vi "LOGGER Loop.vi"(8 "error in":errorcluster, 10 "Queues":T1, 11 "Notifiers":T2) -> (0 "error out":errorcluster)   [LabVIEW 2015, in "Logger.lvlib"]
uses:
  Logger.lvlib
  support/Message Queue/Message Queue.lvlib
  TypeDefs/Logger State.ctl
  TypeDefs/Logger Data.ctl
  Model/TypeDefs/Get Model Status Control.ctl
  Model/Model.lvlib
  <vilib>/ErrorRing/Error Ring.xnode
  support/Global names.vi
  <vilib>/Utility/error.llb/Error Cluster From Error Code.vi
  support/Message Queue/Message Cluster.ctl
  support/Notifiers/Notifiers.ctl
  support/Notifiers/Notifiers.lvlib
  support/Message Queue/All Message Queues.ctl
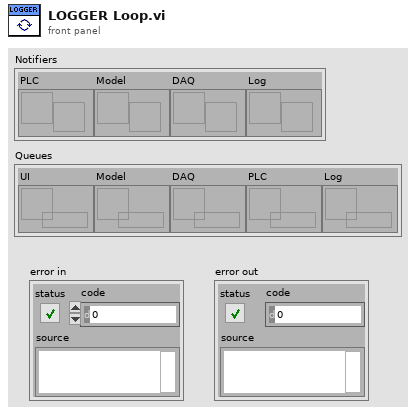
[diagram p1: front panel]
types:
  T1 = typedef "Message Queue.lvlib/All Message Queues.ctl" = cluster{"UI":refnum<queue>, "Model":refnum<queue>, "DAQ":refnum<queue>, "PLC":refnum<queue>, "Log":refnum<queue>}
  T2 = typedef "Notifiers.lvlib/Notifiers.ctl" = cluster{"PLC":refnum<notifier>, "Model":refnum<notifier>, "DAQ":refnum<notifier>, "Log":refnum<notifier>}
  T3 = typedef "Logger.lvlib/Logger Data.ctl" = cluster{"tdms file out":refnum<k34>, "State":T4, "Path":path}
  T4 = typedef "Logger.lvlib/Logger State.ctl" = enum16{"Idle", "Working"}
  T5 = enum16{"open", "open or create", "create or replace", "create", "open (read-only)"}
  T6 = typedef "Model.lvlib/Get Model Status Control.ctl" = cluster{"Position":dbl, "Pump State":bool, "Fluid Flow":dbl, "Fluid Level":dbl, "Barrel Number":i32, "Spill Alarm":bool, "Level Alarm":bool}
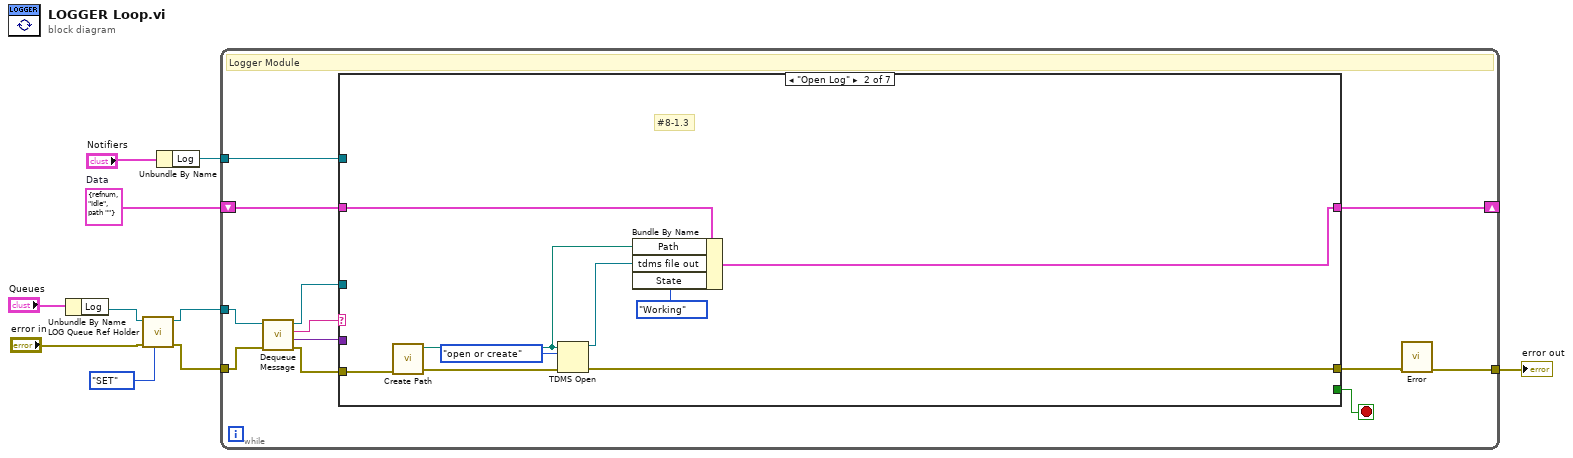
[diagram p0: block diagram]
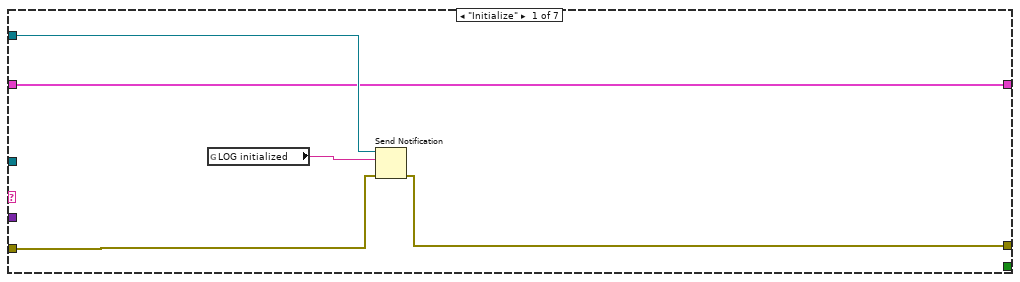
[diagram p2: hidden frame]
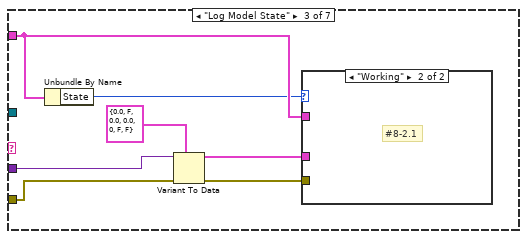
[diagram p3: hidden frame]
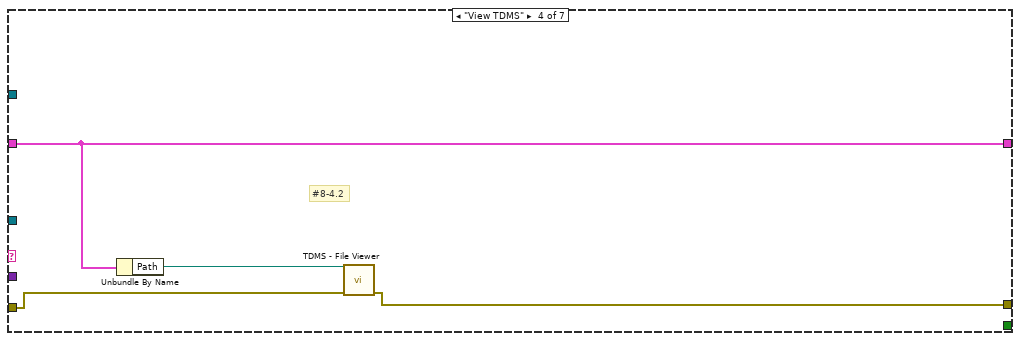
[diagram p5: hidden frame]
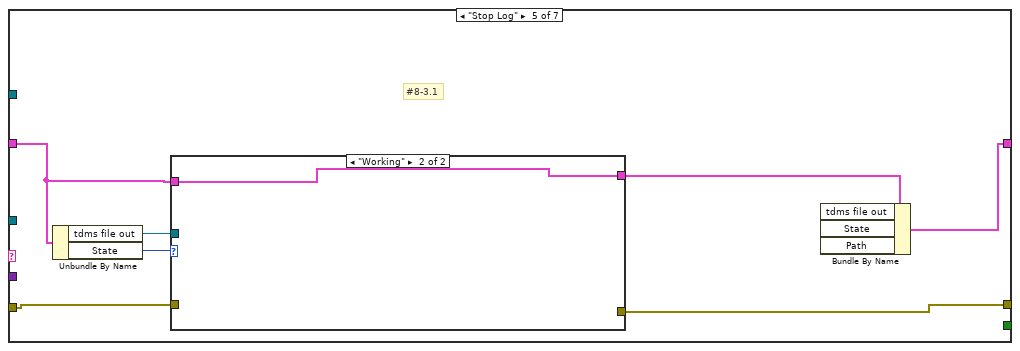
[diagram p6: hidden frame]
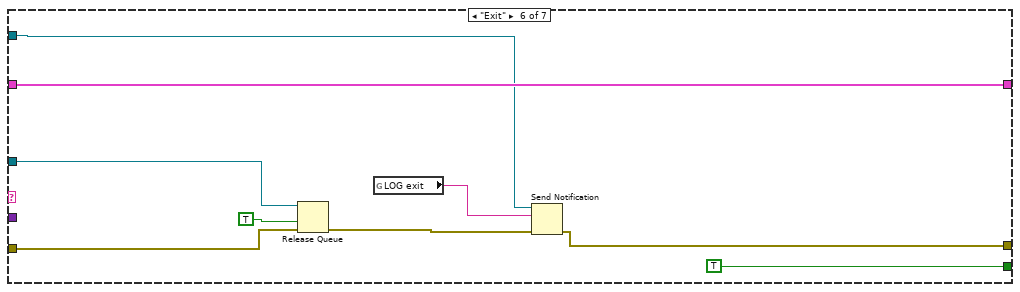
[diagram p8: hidden frame]
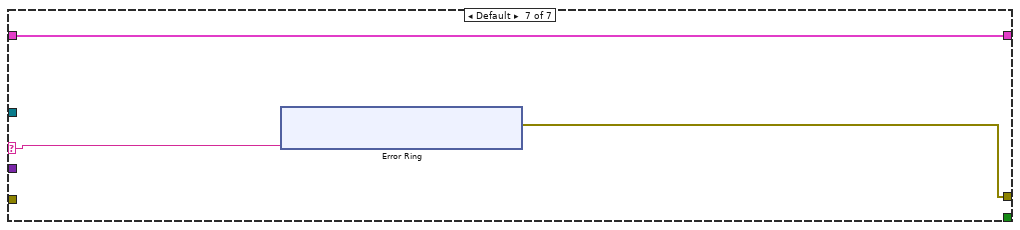
[diagram p9: hidden frame]
diagram:
  w10 = T3 {"tdms file out"=refnum, "State"=enum."Idle", "Path"=path ""}  # Data
  n1 = Unbundle By Name("Queues") -> ("Log"=w3:refnum<queue>)
  n2 = call "LOG Queue Ref Holder.vi"("Action"=enum16{"GET", "SET"}."SET", "error in"="error in", "Message Queue In"=w3) -> ("error out"=w4:errorcluster, "Input Message Queue"=w2:refnum<queue>)  [unwired: 7 in]
  n3 = Unbundle By Name("Notifiers") -> ("Log"=w6:refnum<notifier>)
  n4 = while {
    tunnel: w4 -> [w22]
    tunnel: w2 -> [w21]
    tunnel: [w11] -> w9
    shift-right: [w14] -> _
    shift-left: w10 -> [w15]
    tunnel: w6 -> [w13]
    stop <- w16 stop-if-true
    # "Logger Module"
    n5 = call "Dequeue Message.vi"("error in (no error)"=w22, "Message Queue"=w21) -> ("error out"=w20:errorcluster, "Message Data"=w17:variant, "Message"=w19:string, "dup Message Queue"=w18:refnum<queue>)  [unwired: 6 in]
    n6 = case shown="\"Open Log\"" w19 {
      selector: w19 -> [_ _ _ _ _ _ w68]
      tunnel: w20 -> [w24 w36 w43 w47 w52 w63 _]
      tunnel: w18 -> [_ _ _ _ _ w62 _]
      tunnel: w17 -> [_ _ w41 _ _ _ _]
      tunnel: [w25 w28 _ w45 w48 w64 w67] -> w12
      tunnel: [_ _ _ _ _ TRUE _] -> w16
      tunnel: w15 -> [w26 w33 w38 w46 w50 w66 w69]
      tunnel: [w26 w29 _ w46 w54 w66 w69] -> w14
      tunnel: w13 -> [w27 _ _ _ _ w59 _]
      frame "Initialize" {
        n7 = global read "Global names.vi" "LOG initialized"() -> (w23:string)
        n8 = Send Notification(notification=w23, notifier=w27, error in (no error)=w24) -> (error out=w25:errorcluster)  [unwired: 1 out]
      }
      frame "Open Log" {
        # "#8-1.3"
        n9 = call "Create Path.vi"("error in"=w36) -> ("error out"=w35:errorcluster, "File Path Control"=w30:path)  [unwired: 9 in]
        n10 = TDMS Open(8:w35, 10:T5."open or create" ("operation (0:open)"), 11:w30) -> (0:w28:errorcluster, 3:w31:refnum<k34>)  [unwired: 4 in]
        n11 = Bundle By Name(cluster=w33, "Path"=w30, "tdms file out"=w31, "State"=Logger_State."Working") -> (w29:T3)
      }
      frame "Log Model State" {
        n12 = Unbundle By Name(w38) -> ("State"=w37:T4)
        n13 = Variant To Data(error in=w43, type=T6 {"Position"=0.0, "Pump State"=FALSE, "Fluid Flow"=0.0, "Fluid Level"=0.0, "Barrel Number"=0, "Spill Alarm"=FALSE, "Level Alarm"=FALSE} ("Model Status"), Variant=w41) -> (data=w40:T6, error out=w39:errorcluster)
        n14 = case shown="\"Working\"" w37 {
          tunnel: w40 -> [_ _]
          tunnel: w39 -> [_ _]
          tunnel: w38 -> [_ _]
          frame Default {
          }
          frame "Working" {
            # "#8-2.1"
          }
        }
      }
      frame "View TDMS" {
        # "#8-4.2"
        n15 = Unbundle By Name(w46) -> ("Path"=w44:path)
        n16 = call <vilib>:"TDMS - File Viewer.vi"("error in (no error)"=w47, "file path"=w44) -> ("error out"=w45:errorcluster)  [unwired: 4 in, 1 out]
      }
      frame "Stop Log" {
        # "#8-3.1"
        n17 = Unbundle By Name(w50) -> ("tdms file out"=w53:refnum<k34>, "State"=w51:T4)
        n18 = case shown="\"Working\"" w51 {
          tunnel: w53 -> [_ _]
          tunnel: w52 -> [w56 _]
          tunnel: [w56 _] -> w48
          tunnel: w50 -> [w55 w57]
          tunnel: [w55 w57] -> w49
          frame "Idle", Default {
          }
          frame "Working" {
          }
        }
        n19 = Bundle By Name(cluster=w49) -> (w54:T3)  [unwired: 3 in]
      }
      frame "Exit" {
        n20 = Release Queue(queue=w62, force destroy? (F)=TRUE, error in (no error)=w63) -> (error out=w61:errorcluster)  [unwired: 2 out]
        n21 = global read "Global names.vi" "LOG exit"() -> (w58:string)
        n22 = Send Notification(notification=w58, notifier=w59, error in (no error)=w61) -> (error out=w64:errorcluster)  [unwired: 1 out]
      }
      frame Default {
        n23 = xnode "Error Ring"("parameter 0"=w68) -> ("error out"=w67:errorcluster)
      }
    }
    n24 = call "Error.vi"("error in"=w12) -> ("error out"=w11:errorcluster)  [unwired: 10 in]
  }
  "error out" <- w9
